vi "Counter Open.vi"(8 "error in":errorcluster, 9 "Reset (True)":bool=TRUE, 10 "ID Query (True)":bool=TRUE, 11 "couner session in":T1) -> (0 "error out":errorcluster, 2 "idn string":string, 3 "counter session out":T1)   [LabVIEW 2020, in "Counter.lvlib"]
doc: "Opens counter session."
uses:
  Counter.lvlib
  Counter Session.ctl
  Counter Type.ctl
  Picotest U62XXA/PICOTEST U62XXA series.lvlib
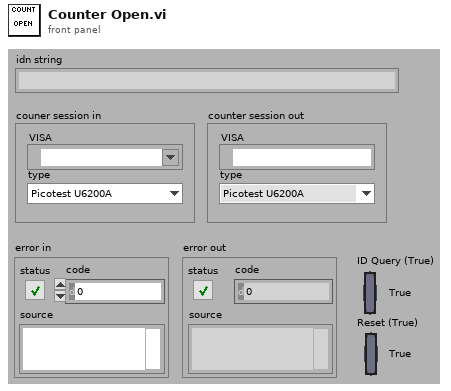
[diagram p1: front panel]
types:
  T1 = typedef "Counter.lvlib/Counter Session.ctl" = cluster{"VISA":refnum<visa-resource-name>, "type":T2}
  T2 = typedef "Counter.lvlib/Counter Type.ctl" = enum16{"Picotest U6200A", "dummy"}
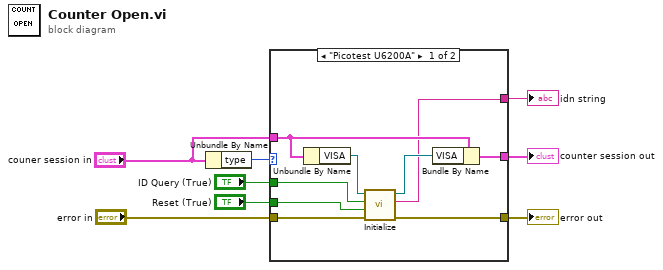
[diagram p0: block diagram]
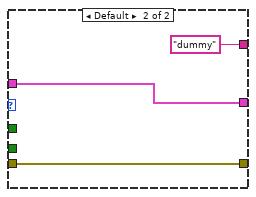
[diagram p2: hidden frame]
diagram:
  n1 = Unbundle By Name("couner session in") -> ("type"=w8:T2)
  n2 = case shown="\"Picotest U6200A\"" w8 {
    tunnel: "error in" -> [w17 w20]
    tunnel: "couner session in" -> [w14 w19]
    tunnel: [w13 w20] -> w6
    tunnel: [w12 w19] -> w3
    tunnel: [w11 "dummy" ("idn string")] -> w5
    tunnel: "ID Query (True)" -> [w10 _]
    tunnel: "Reset (True)" -> [w9 _]
    frame "Picotest U6200A" {
      n3 = Unbundle By Name(w14) -> ("VISA"=w16:refnum<visa-resource-name>)
      n4 = call "Initialize.vi"("error in (no error)"=w17, "Reset (True)"=w9, "ID Query (True)"=w10, "VISA resource name"=w16) -> ("error out"=w13:errorcluster, "idn string"=w11:string, "VISA resource name out"=w15:refnum<visa-resource-name>)  [unwired: 5 in]
      n5 = Bundle By Name(cluster=w14, "VISA"=w15) -> (w12:T1)
    }
    frame Default {
    }
  }
  "error out" <- w6
  "counter session out" <- w3
  "idn string" <- w5
